vi "WriteToFile.vi"(7 "Write to file":bool, 8 "error in":errorcluster, 9 "sub folder":string="runs", 10 "Output File":string, 11 "contents":string) -> (2 "error out":errorcluster, 3 "path":path)   [LabVIEW 2017]
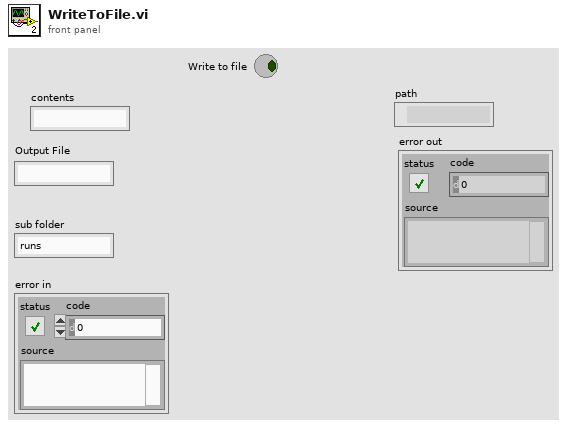
[diagram p1: front panel]
types:
  T1 = enum16{"open", "replace", "create", "open or create", "replace or create", "replace or create with confirmation"}
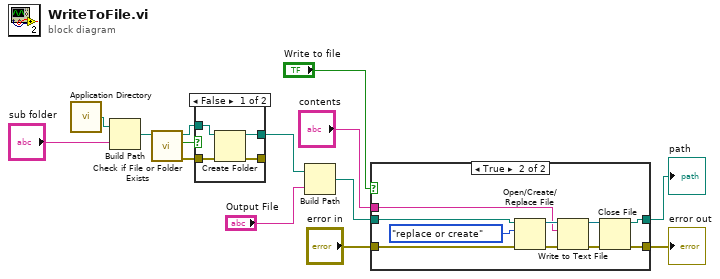
[diagram p0: block diagram]
diagram:
  n1 = call <vilib>:"Application Directory.vi"() -> ("Application Directory"=w10:path)
  n2 = Build Path(base path=w10, name or relative path="sub folder") -> (appended path=w6:path)
  n3 = call <vilib>:"Check if File or Folder Exists.vi"("path"=w6) -> ("error out"=w7:errorcluster, "file or folder exists?"=w8:bool, "dup path"=w9:path)  [unwired: 8 in]
  n4 = case shown="False" w8 {
    tunnel: w9 -> [w18 w20]
    tunnel: [w17 w20] -> w14
    tunnel: w7 -> [w16 w19]
    tunnel: [w15 w19] -> _
    frame False {
      n5 = Create Folder(path (use dialog)=w18, error in=w16) -> (created path=w17:path, error out=w15:errorcluster)  [unwired: 1 in, 1 out]
    }
    frame True {
    }
  }
  n6 = Build Path(base path=w14, name or relative path="Output File") -> (appended path=w12:path)
  n7 = case shown="True" "Write to file" {
    tunnel: w12 -> [w21 w28]
    tunnel: [w21 w26] -> w5
    tunnel: [w22 w25] -> w4
    tunnel: "error in" -> [w22 w24]
    tunnel: "contents" -> [_ w23]
    frame False {
    }
    frame True {
      n8 = Open/Create/Replace File(file path (use dialog)=w28, error in=w24, operation (0:open)=T1."replace or create") -> (refnum out=w32:refnum<file>, error out=w29:errorcluster)  [unwired: 3 in, 1 out]
      n9 = Write to Text File(file (use dialog)=w32, text=w23, error in=w29) -> (refnum out=w31:refnum<file>, error out=w30:errorcluster)  [unwired: 1 in, 1 out]
      n10 = Close File(refnum=w31, error in=w30) -> (path=w26:path, error out=w25:errorcluster)
    }
  }
  "path" <- w5
  "error out" <- w4
